vi "DriveJoystickAcquire.vi"(8 "Rotation Joystick Deadband %":dbl, 11 "XY Joystick Deadband %":dbl) -> (0 "Drive Joystick Buttons":bool[](array[boolean]), 2 "Joystick Data":T1, 3 "Drive Joystick Values":dbl[](array[numeric]))   [LabVIEW 2019]
uses:
  Controls/DriveJoystickData.ctl
  <vilib>/Rock Robotics/WPI/Utilities/WPI_GetSetVariantRefNum.vi
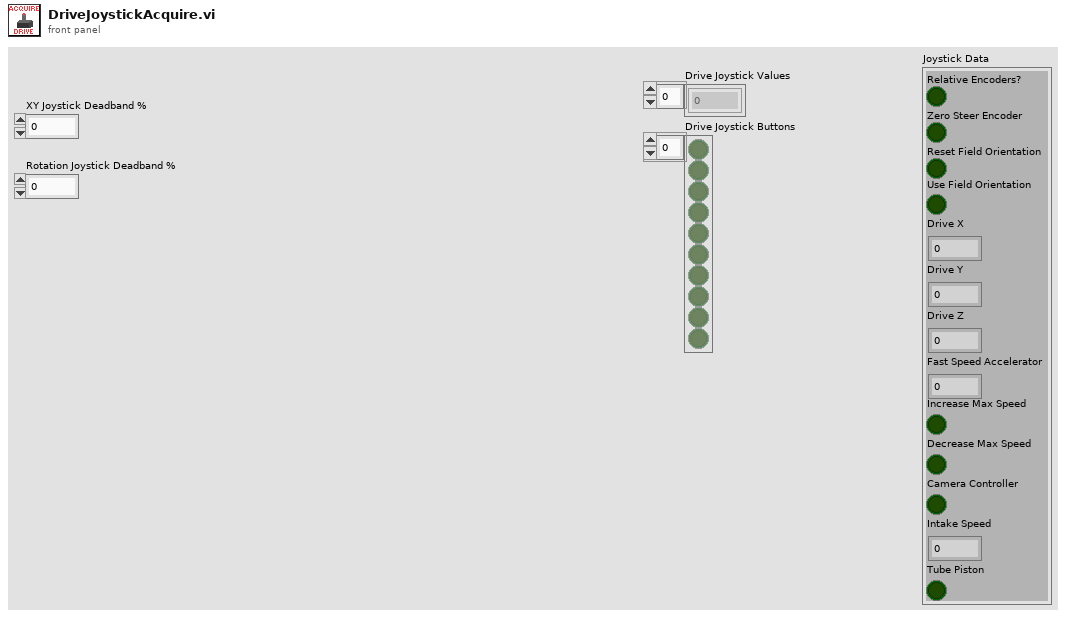
[diagram p1: front panel]
types:
  T1 = typedef "DriveJoystickData.ctl" = cluster{"Relative Encoders?":bool, "Zero Steer Encoder":bool, "Reset Field Orientation":bool, "Use Field Orientation":bool, "Drive X":dbl, "Drive Y":dbl, "Drive Z":dbl, "Fast Speed Accelerator":dbl, "Increase Max Speed":bool, "Decrease Max Speed":bool, "Camera Controller":bool, "Intake Speed":dbl, "Tube Piston":bool}
  T2 = typedef "WPI_JoystickDevRef.ctl" = cluster{"Device":T3}
  T3 = typedef "WPI_JoystickDeviceEnum.ctl" = enum16{"USB 0", "USB 1", "USB 2", "USB 3", "USB 4", "USB 5"}
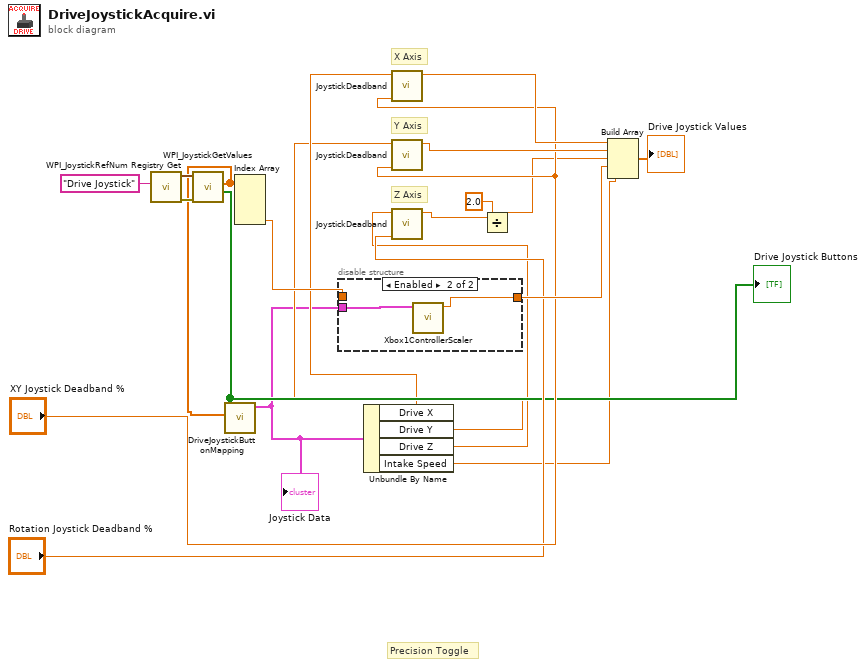
[diagram p0: block diagram]
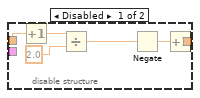
[diagram p2: hidden frame]
diagram:
  # "Precision Toggle"
  # "Z Axis"
  # "Y Axis"
  # "X Axis"
  n1 = call <vilib>:"WPI_JoystickRefNum Registry Get.vi"("refnum name"="Drive Joystick") -> ("error out"=w20:errorcluster, "JoystickDevRef"=w19:T2)  [unwired: 9 in]
  n2 = call <vilib>:"WPI_JoystickGetValues.vi"("error in (no error)"=w20, "JoystickDevRef"=w19) -> ("Buttons"=w10:bool[], "Axes"=w2:dbl[])  [unwired: 5 in, 3 out]
  "Drive Joystick Buttons" <- w10
  n3 = call "DriveJoystickButtonMapping.vi"("Joystick Values"=w2, "drive joystick buttons"=w10) -> ("output cluster"=w3:T1)  [unwired: 8 in, 1 out]
  "Joystick Data" <- w3
  n4 = Index Array(array=w2) -> (element #4=w17:dbl)  [unwired: 4 in, 3 out]
  n5 = disable-structure shown="Enabled" {
    disable-tunnel: w17 -> [w24 _]
    disable-tunnel: [w21 w27] -> w16
    disable-tunnel: w3 -> [_ w28]
    frame Disabled {
      n6 = Increment(x=w24) -> (x+1=w25:dbl)
      n7 = Divide(x=w25, y=2.0) -> (x/y=w23:dbl)
      n8 = Negate(x=w23) -> (-x=w22:dbl)
      n9 = Increment(x=w22) -> (x+1=w21:dbl)
    }
    frame Enabled {
      n10 = call "Xbox1ControllerScaler.vi"("DriveJoystickButtonMapping"=w28) -> ("Speed"=w27:dbl)  [unwired: 10 in]
    }
  }
  n11 = Unbundle By Name(w3) -> ("Drive X"=w6:dbl, "Drive Y"=w5:dbl, "Drive Z"=w4:dbl, "Intake Speed"=w1:dbl)
  n12 = call "JoystickDeadband.vi"("Deadband %"="XY Joystick Deadband %", "Joystick Value"=w6) -> ("Joystick Value"=w14:dbl)  [unwired: 9 in]
  n13 = call "JoystickDeadband.vi"("Deadband %"="XY Joystick Deadband %", "Joystick Value"=w5) -> ("Joystick Value"=w15:dbl)  [unwired: 9 in]
  n14 = call "JoystickDeadband.vi"("Deadband %"="Rotation Joystick Deadband %", "Joystick Value"=w4) -> ("Joystick Value"=w8:dbl)  [unwired: 9 in]
  n15 = Divide(x=w8, y=2.0) -> (x/y=w9:dbl)
  n16 = Build Array(w14, w15, w9, w16, w1) -> (→"Drive Joystick Values":dbl[])
